vi "Initialise session.vi"(7 "Node ID":u8 min=1 max=127 step=1, 8 "error in":errorcluster, 10 "Motor":u8(ring) items=["Right", "Left"]) -> (0 "error out":errorcluster, 3 "interface object out":refnum<k20>, 5 "Used Node ID":u8 min=1 max=127 step=1)   [LabVIEW 2016]
uses:
  Motor controllers.vi
  <vilib>/CANopenLib/CANOPEN.llb/CANopen Interface Create.vi
  <vilib>/CANopenLib/CANOPEN.llb/CANopen SDO Create.vi
  <vilib>/CANopenLib/CANOPEN.llb/CANopen SDO Close.vi
panel:
  # "If zero use default"
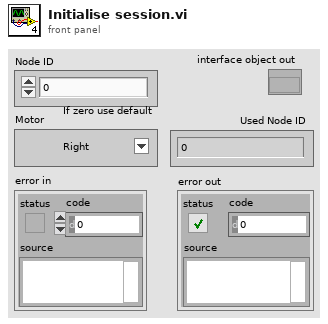
[diagram p1: front panel]
types:
  T1 = cluster{"termination resistor":bool, "CANopen interface":u32, "baud rate":u32, "FPGA VI Reference":refnum<k20>, "interface object out":refnum<k20>}
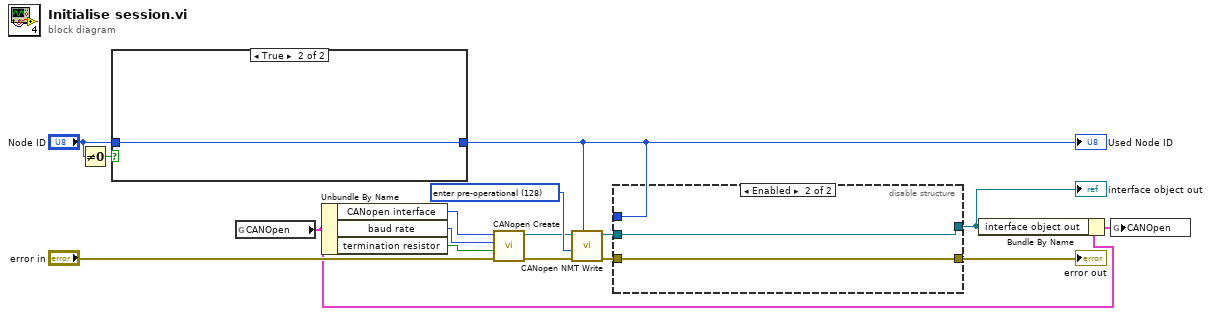
[diagram p0: block diagram]
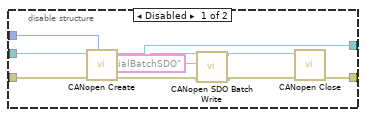
[diagram p2: hidden frame]
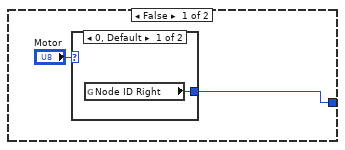
[diagram p3: hidden frame]
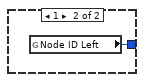
[diagram p4: hidden frame]
diagram:
  w16 = u16 128 items=["start remote node"=1, "stop remote node"=2, "enter pre-operational"=128, "reset node"=129, "reset communication"=130] ("command")
  n1 = Not Equal To 0?(x="Node ID") -> (x != 0?=w9:bool)
  n2 = case shown="True" w9 {
    tunnel: [w17 w21] -> w3
    tunnel: "Node ID" -> [_ w21]
    frame False {
      n3 = case shown="0, Default" "Motor" {
        tunnel: [w19 w20] -> w17
        frame 0, Default {
          n4 = global read "Motor controllers.vi" "Node ID Right"() -> (w19:u8)
        }
        frame 1 {
          n5 = global read "Motor controllers.vi" "Node ID Left"() -> (w20:u8)
        }
      }
    }
    frame True {
    }
  }
  "Used Node ID" <- w3
  n6 = global read "Motor controllers.vi" "CANOpen"() -> (w7:T1)
  n7 = Unbundle By Name(w7) -> ("CANopen interface"=w12:u32, "baud rate"=w11:u32, "termination resistor"=w10:bool)
  n8 = call-poly <vilib>:"CANopen Create.vi"("error in (no error)"="error in", "termination? (F)"=w10, "baud rate"=w11, "interface name"=w12) -> ("error out"=w13:errorcluster, "interface object out"=w14:refnum<k20>)  [unwired: 6 in]
  n9 = call <vilib>:"CANopen NMT Write.vi"("node-ID (0)"=w3, "error in (no error)"=w13, "command"=w16, "interface object in"=w14) -> ("error out"=w5:errorcluster, "interface object out"=w4:refnum<k20>)  [unwired: 6 in]
  n10 = disable-structure shown="Enabled" {
    disable-tunnel: w5 -> [w31 w33]
    disable-tunnel: w4 -> [w30 w32]
    disable-tunnel: w3 -> [w29 _]
    disable-tunnel: [w28 w33] -> w2
    disable-tunnel: [w27 w32] -> w1
    frame Disabled {
      n11 = call-poly <vilib>:"CANopen Create.vi"("node-ID"=w29, "error in (no error)"=w31, "interface object in"=w30) -> ("error out"=w25:errorcluster, "SDO object out"=w26:refnum<k20>, "interface object out"=w27:refnum<k20>)  [unwired: 6 in]
      n12 = call <vilib>:"CANopen SDO Batch Write.vi"("error in (no error)"=w25, "batch SDO name"="InitialBatchSDO", "SDO object in"=w26) -> ("error out"=w24:errorcluster, "SDO object out"=w23:refnum<k20>)  [unwired: 6 in, 1 out]
      n13 = call-poly <vilib>:"CANopen Close.vi"("error in (no error)"=w24, "SDO object in"=w23) -> ("error out"=w28:errorcluster)  [unwired: 9 in]
    }
    frame Enabled {
    }
  }
  "error out" <- w2
  "interface object out" <- w1
  n14 = Bundle By Name(cluster=w7, "interface object out"=w1) -> (w6:T1)
  n15 = global write "Motor controllers.vi" "CANOpen"(w6) -> ()
